vi "pH_所有参数读取.vi"(8 "error in (no error)":errorcluster caption="错误输入（无错误）", 11 "MB_Serial session in":refnum<class "MB_Master_Serial.lvclass">) -> (0 "error out":errorcluster caption="错误输出", 2 "输出值":T1 {"电极型号标志" items=["NULL", "pH", "Cond", "DO", "Turb"]; "电极状态标志" items=["OK", "第一点校正通过", "第二点校正通过", "校正失败,电极零点超出范围", "校正失败,电极斜率超出范围", "第三点校正通过"]}, 3 "MB_Serial session out":refnum<class "MB_Master_Serial.lvclass">)   [LabVIEW 2016, in "斯坦道多参数.lvlib"]
uses:
  <vilib>/Plasmionique/MB Master/MB_Master_Serial/MB_Master_Serial.lvclass
  C:/Program Files (x86)/National Instruments/LabVIEW 2016/vi.lib/Plasmionique/MB Master/MB_Master/MB_Master.lvclass
  <vilib>/Plasmionique/MB Master/MB Master.lvlib
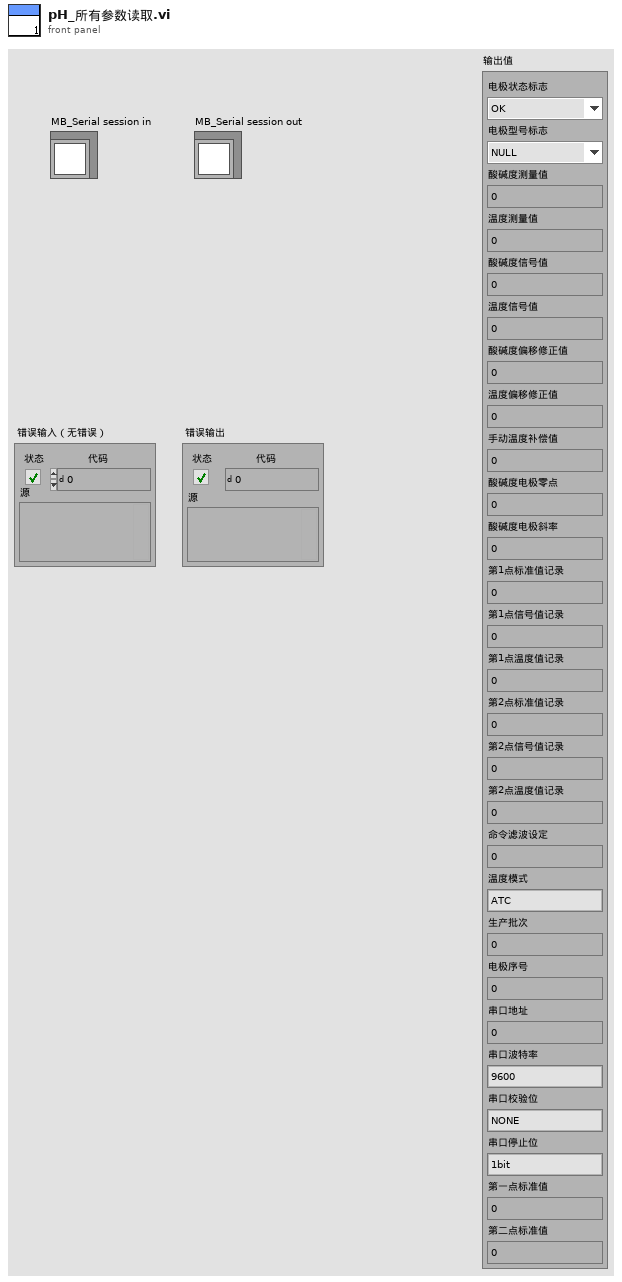
[diagram p1: front panel]
types:
  T1 = cluster{"电极状态标志":u16, "电极型号标志":u16, "酸碱度测量值":sgl, "温度测量值":sgl, "酸碱度信号值":sgl, "温度信号值":sgl, "酸碱度偏移修正值":sgl, "温度偏移修正值":sgl, "手动温度补偿值":sgl, "酸碱度电极零点":sgl, "酸碱度电极斜率":sgl, "第1点标准值记录":sgl, "第1点信号值记录":sgl, "第1点温度值记录":sgl, "第2点标准值记录":sgl, "第2点信号值记录":sgl, "第2点温度值记录":sgl, "命令滤波设定":u16, "温度模式":enum16{"ATC", "MTC"}, "生产批次":u16, "电极序号":u16, "串口地址":u16, "串口波特率":enum16{"9600", "19200", "115200"}, "串口校验位":enum16{"NONE", "ODD", "EVEN"}, "串口停止位":enum16{"1bit", "2bit"}, "第一点标准值":sgl, "第二点标准值":sgl}
  T2 = cluster{u16, u16, "数值":sgl, "数值":sgl, "数值":sgl, "数值":sgl, "数值":sgl, "数值":sgl, "数值":sgl, "数值":sgl, "数值":sgl, "数值":sgl, "数值":sgl, "数值":sgl, "数值":sgl, "数值":sgl, "数值":sgl, u16, u16, u16, u16, u16, u16, u16, u16, "数值":sgl, "数值":sgl}
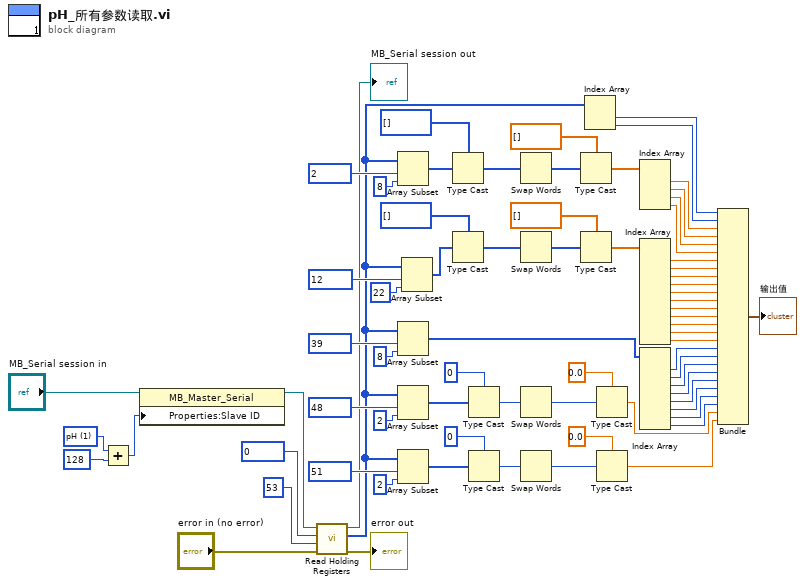
[diagram p0: block diagram]
diagram:
  w72 = u16 1 items=["NULL", "pH", "Cond", "DO", "Turb"] ("数值")
  n1 = Add(x=w72, y=u16 128) -> (x+y=w70:u16)
  n2 = property class="MB_Master_Serial"(reference="MB_Serial session in", "Properties:Slave ID"=w70) -> (reference out=w4:refnum<class "MB_Master_Serial.lvclass">)  [unwired: 1 in, 1 out]
  n3 = call <vilib>:"Read Holding Registers.vi"("error in (no error)"="error in (no error)", "quantity"=u16 53, "starting address"=u16 0, "MB session in"=w4) -> ("error out"=→"error out":errorcluster, "Registers"=w18:u16[], "MB session out"=→"MB_Serial session out":refnum<class "MB_Master_Serial.lvclass">)  [unwired: 5 in]
  n4 = Array Subset(array=w18, index=u16 2 ("starting address"), length=8 ("长度")) -> (w59:u16[])
  n5 = Array Subset(array=w18, index=u16 39 ("starting address"), length=8 ("长度")) -> (w31:u16[])
  n6 = Array Subset(array=w18, index=u16 48 ("starting address"), length=2 ("长度")) -> (w13:u16[])
  n7 = Array Subset(array=w18, index=u16 51 ("starting address"), length=2 ("长度")) -> (w8:u16[])
  n8 = Array Subset(array=w18, index=u16 12 ("starting address"), length=22 ("长度")) -> (w48:u16[])
  n9 = Type Cast(type=u32[] [] ("数组 2"), x=w59) -> (*(type *) &x=w61:u32[])
  n10 = Type Cast(type=u32[] [] ("数组 2"), x=w48) -> (*(type *) &x=w51:u32[])
  n11 = Type Cast(type=u32 0 ("数值"), x=w13) -> (*(type *) &x=w16:u32)
  n12 = Type Cast(type=u32 0 ("数值"), x=w8) -> (*(type *) &x=w10:u32)
  n13 = Swap Words(1:w61) -> (0:w63:u32[])
  n14 = Swap Words(1:w51) -> (0:w52:u32[])
  n15 = Swap Words(1:w16) -> (0:w17:u32)
  n16 = Swap Words(1:w10) -> (0:w9:u32)
  n17 = Type Cast(type=sgl[] [] ("数组 2"), x=w63) -> (*(type *) &x=w58:sgl[])
  n18 = Type Cast(type=sgl[] [] ("数组 2"), x=w52) -> (*(type *) &x=w47:sgl[])
  n19 = Index Array(array=w18) -> (element #1=w66:u16, element #2=w65:u16)  [unwired: 2 in]
  n20 = Type Cast(type=sgl 0.0 ("数值"), x=w17) -> (*(type *) &x=w7:sgl)
  n21 = Type Cast(type=sgl 0.0 ("数值"), x=w9) -> (*(type *) &x=w6:sgl)
  n22 = Index Array(array=w58) -> (element #1=w57:sgl, element #2=w56:sgl, element #3=w55:sgl, element #4=w54:sgl)  [unwired: 4 in]
  n23 = Index Array(array=w47) -> (element #1=w46:sgl, element #2=w45:sgl, element #3=w44:sgl, element #4=w43:sgl, element #5=w42:sgl, element #6=w41:sgl, element #7=w40:sgl, element #8=w39:sgl, element #9=w38:sgl, element #10=w37:sgl, element #11=w36:sgl)  [unwired: 11 in]
  n24 = Index Array(array=w31) -> (element #1=w30:u16, element #2=w29:u16, element #3=w28:u16, element #4=w27:u16, element #5=w26:u16, element #6=w25:u16, element #7=w24:u16, element #8=w23:u16)  [unwired: 8 in]
  n25 = Bundle(w66, w65, "数值"=w57, "数值"=w56, "数值"=w55, "数值"=w54, "数值"=w46, "数值"=w45, "数值"=w44, "数值"=w43, "数值"=w42, "数值"=w41, "数值"=w40, "数值"=w39, "数值"=w38, "数值"=w37, "数值"=w36, w30, w29, w28, w27, w26, w25, w24, w23, "数值"=w7, "数值"=w6) -> (→"输出值":T2)  [unwired: 1 in]
